vi "Initial State Example - Looping.vi"() -> ()   [LabVIEW 2013]
doc: "This example sends random data to your Initial State accout. To use this example first create an Initial State account for free at www.initialstate.com. Once created place your access key in the associated field and hit run."
uses:
  Controls/IS Data Point TypeDef (String).ctl
  Data Helpers/IS PolyVI Instance Bool To JSON Cluster .vi
  Data Helpers/IS PolyVI Instance String to JSON Cluster.vi
  Data Helpers/IS PolyVI Instance DBL To JSON Cluster .vi
panel:
  out "Buffer Size":i32
  in  "stop":bool
  out "Waveform Chart":dbl(graph)=0.6082396240250167
  in  "Bucket Name (Optional)":string="LabVIEW Example Bucket"
  in  "Access Key":string="FakeFakeVj0GLMeSHRkyOEAPFGhzWEmw"
  out "Response Headers":string
  out "Response Body":string
  # "Initial State Streaming LabVIEW Example"
  # "To use this example first create an Initial State account for free at www.initialstate.com. Once created place your access key in the associated field below and hit run."
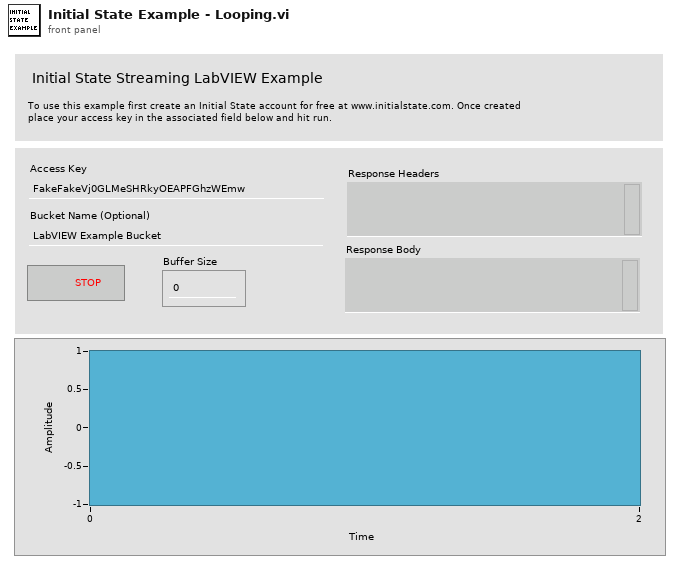
[diagram p1: front panel]
types:
  T1 = typedef "IS Data Point TypeDef (String).ctl" = cluster{"key":string, "value":string, "epoch":dbl}
  T2 = typedef "IS Session.ctl" = cluster{"Access Key":string, "HTTP Client Handle":T3}
  T3 = typedef "LabVIEWHTTPClient.lvlib/ClientHandle.ctl" = refnum<k1>
  T4 = typedef "IS Bucket Session.ctl" = cluster{"Bucket Key":string}
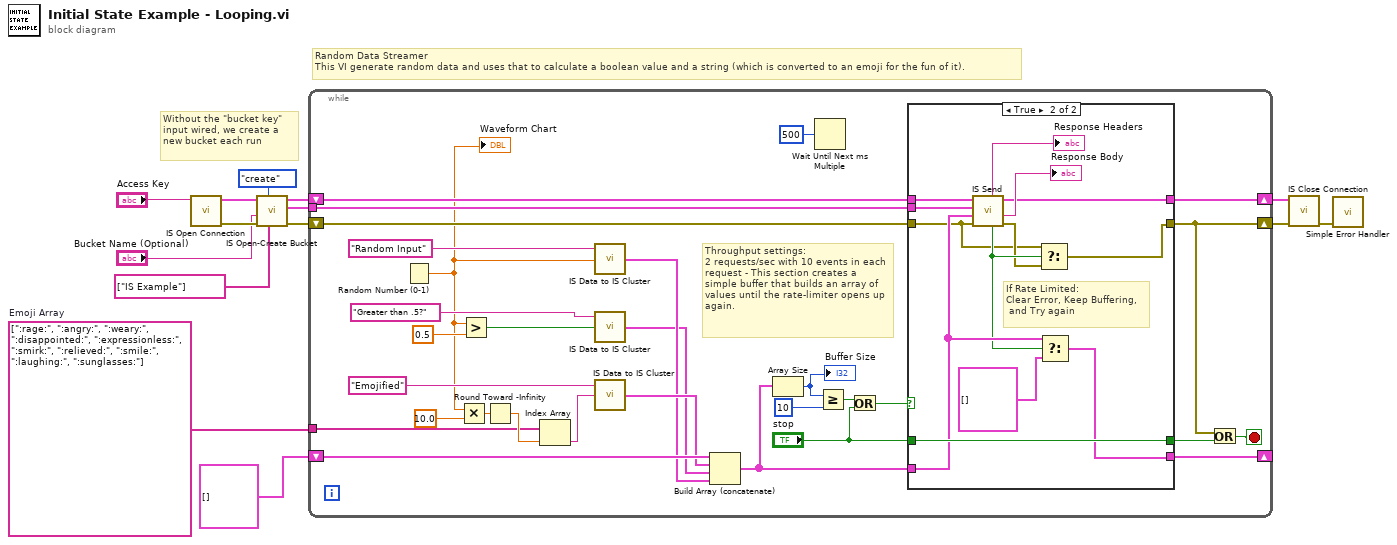
[diagram p0: block diagram]
diagram:
  w5 = string[] [":rage:", ":angry:", ":weary:", ":disappointed:", ":expressionless:", ":smirk:", ":relieved:", ":smile:", ":laughing:", ":sunglasses:"]  # Emoji Array
  # "Without the \"bucket key\" input wired, we create a new bucket each run"
  # "Random Data Streamer\nThis VI generate random data and uses that to calculate a boolean value and a string (which is converted to an emoji for the fun of it)."
  n1 = call "IS Open Connection.vi"("Access Key"="Access Key") -> ("error out"=w12:errorcluster, "IS Session"=w14:T2)  [unwired: 9 in]
  n2 = call "IS Open-Create Bucket.vi"("Tags (Optional: Auto-Populates \"labview\")"=string[] ["IS Example"] ("Tags (Optional: Auto-Populates \"labview\")"), "Operation (0: open)"=enum16{"open", "create"}."create", "error in (no error)"=w12, "Bucket Name (Optional)"="Bucket Name (Optional)", "IS Session In"=w14) -> ("error IO"=w6:errorcluster, "IS Bucket Session"=w9:T4, "IS Session Out"=w8:T2)  [unwired: 4 in]
  n3 = while {
    tunnel: w9 -> [w41]
    shift-right: [w44] -> w4
    shift-left: w8 -> [w43]
    shift-right: [w24] -> w3
    shift-left: w6 -> [w42]
    shift-right: [w39] -> _
    shift-left: T1[] [] -> [w40]
    tunnel: w5 -> [w29]
    stop <- w23 stop-if-true
    # "Throughput settings: \n2 requests/sec with 10 events in each request - This section creates a simple buffer that builds an array of values until the rate-limiter opens up again."
    n4 = Random Number (0-1)() -> (number: 0 to 1=w18:dbl)
    "Waveform Chart" <- w18
    n5 = Multiply(x=w18, y=10.0) -> (x*y=w32:dbl)
    n6 = Greater?(x=w18, y=0.5) -> (0:w17:bool)
    n7 = Round Toward -Infinity(1:w32) -> (0:w30:dbl)
    n8 = Index Array(array=w29, index=w30) -> (element=w16:string)
    n9 = call-poly "IS Data to IS Cluster.vi"("Stream Value"=w18, "Stream Key"="Random Input") -> ("JSON Cluster Array out"=w26:T1[])  [unwired: 3 in]
    n10 = call-poly "IS Data to IS Cluster.vi"("Stream Value"=w17, "Stream Key"="Greater than .5?") -> ("JSON Cluster Array out"=w25:T1[])  [unwired: 3 in]
    n11 = call-poly "IS Data to IS Cluster.vi"("Stream Value"=w16, "Stream Key"="Emojified") -> ("JSON Cluster Array out"=w27:T1[])  [unwired: 3 in]
    n12 = Build Array (concatenate)(w40, w27, w25, w26) -> (w38:T1[])
    n13 = Array Size(array=w38) -> (size(s)=w37:i32)
    "Buffer Size" <- w37
    n14 = Wait Until Next ms Multiple(millisecond multiple=u32 500) -> ()  [unwired: 1 out]
    n15 = Greater Or Equal?(x=w37, y=10) -> (x >= y?=w21:bool)
    n16 = Or(x=w21, y="stop") -> (x .or. y?=w20:bool)
    n17 = case shown="True" w20 {
      tunnel: [w48 w57] -> w44
      tunnel: [w47 w49] -> w24
      tunnel: w43 -> [w48 w61]
      tunnel: w42 -> [w47 w50]
      tunnel: w41 -> [_ w60]
      tunnel: w38 -> [w46 w54]
      tunnel: [w46 w53] -> w39
      tunnel: "stop" -> [w45 w58]
      tunnel: [w45 w58] -> w22
      frame False {
      }
      frame True {
        # "If Rate Limited: \nClear Error, Keep Buffering,\n and Try again"
        n18 = call "IS Send.vi"("error in (no error)"=w50, "JSON Custer Array in"=w54, "IS Bucket Session"=w60, "IS Session in"=w61) -> ("Error out"=w51:errorcluster, "Response Body"=→"Response Body":string, "IS Session out"=w57:T2, "Rate Limit Reached?"=w52:bool, "Response Headers"=→"Response Headers":string)  [unwired: 2 in, 1 out]
        n19 = Select(t=w50, s=w52, f=w51) -> (s? t:f=w49:errorcluster)
        n20 = Select(t=w54, s=w52, f=T1[] []) -> (s? t:f=w53:T1[])
      }
    }
    n21 = Or(x=w24, y=w22) -> (x .or. y?=w23:bool)
  }
  n22 = call "IS Close Connection.vi"("error in (no error)"=w3, "IS Session In"=w4) -> ("error out"=w11:errorcluster)  [unwired: 9 in]
  n23 = call <vilib>:"Simple Error Handler.vi"("error in (no error)"=w11) -> ()  [unwired: 4 in, 5 out]
